vi "build_string_activity22.vi"() -> ()   [LabVIEW 2025]
panel:
  out "Length of string":dbl
  out "Combined string":string
  in  "Trailer":string
  in  "Number":sgl
  in  "Header":string
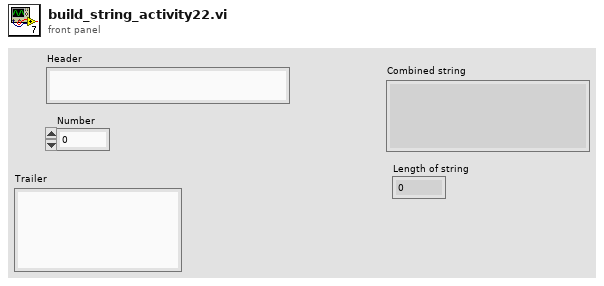
[diagram p1: front panel]
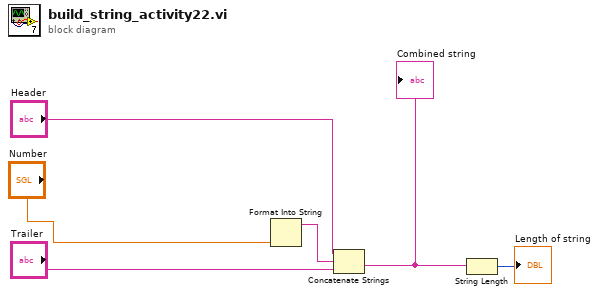
[diagram p0: block diagram]
diagram:
  n1 = Format Into String("Number") -> (resulting string=w2:string)  [unwired: 3 in, 1 out]
  n2 = Concatenate Strings("Header", w2, "Trailer") -> (w1:string)
  "Combined string" <- w1
  n3 = String Length(string=w1) -> (length=→"Length of string":i32)
